vi "InitDone.vi"(8 "error in (no error)":errorcluster, 11 "TranslationStageActor in":refnum<class "ArduinoTranslationStage.lvclass">) -> (0 "error out":errorcluster, 3 "TranslationStageActor out":refnum<class "ArduinoTranslationStage.lvclass">)   [LabVIEW 2023]
uses:
  ArduinoTranslationStage.lvclass
  ArduinoTranslationStage.lvclass/ArduinoTranslationStage.ctl
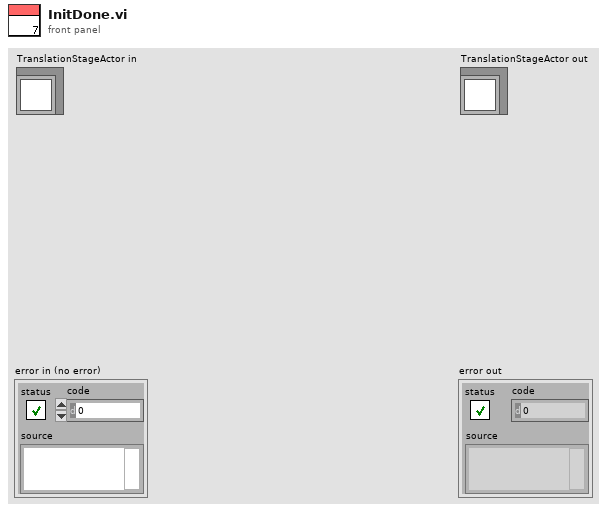
[diagram p1: front panel]
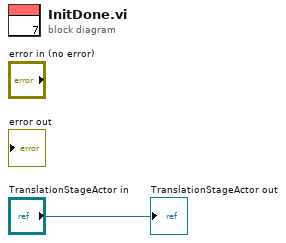
[diagram p0: block diagram]
diagram:
  "TranslationStageActor out" <- "TranslationStageActor in"
